vi "Pcre2NextMatch8.vi"(8 "error in":errorcluster, 11 "pMatchData":u64 format="%.0x") -> (0 "error out":errorcluster, 1 "GlobalOptions":u32 format="%.0x", 2 "NextStartOffset":u64, 3 "pMatchData":u64 format="%.0x", 5 "ContinueMatch?":bool)   [LabVIEW 2021, in "libpcre2-8.lvlib"]
uses:
  libpcre2-8.lvlib
  libpcre2-8-x32.dll
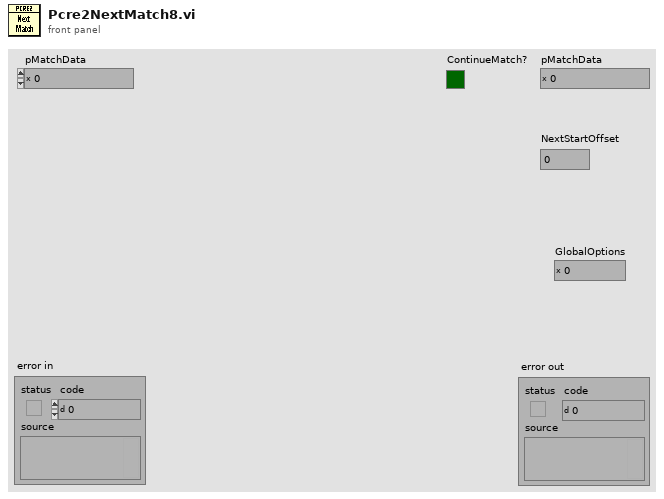
[diagram p1: front panel]
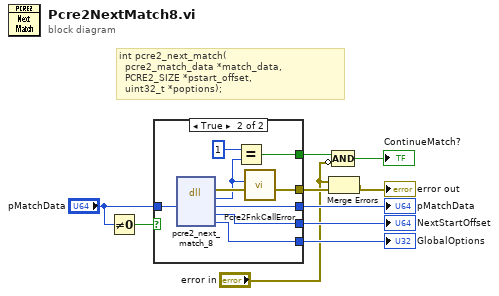
[diagram p0: block diagram]
diagram:
  # "int pcre2_next_match(\n  pcre2_match_data *match_data, \n  PCRE2_SIZE *pstart_offset, \n  uint32_t *poptions);"
  n1 = Not Equal To 0?(x="pMatchData") -> (x != 0?=w6:bool)
  n2 = case shown="True" w6 {
    tunnel: [_ w19] -> w3
    tunnel: "pMatchData" -> [_ w17]
    tunnel: [_ w16] -> w10
    tunnel: [_ w13] -> w5
    tunnel: [_ w12] -> w9
    tunnel: [_ w11] -> w8
    frame False {
    }
    frame True {
      n3 = dll-call lib="libpcre2-8-x*.dll" fn="pcre2_next_match_8"("match_data"=w17) -> (error out=w18:errorcluster, "result"=w15:i32, "match_data"=w16:u64, "pstart_offset"=w12:u64, "poptions"=w11:u32)  [unwired: 5 in, 1 out]
      n4 = Equal?(x=1, y=w15) -> (x = y?=w13:bool)
      n5 = call "Pcre2FnkCallError.vi"("error in"=w18, "ErrorCode"=w15) -> ("error out"=w19:errorcluster)  [unwired: 9 in]
    }
  }
  "pMatchData" <- w10
  "NextStartOffset" <- w9
  "GlobalOptions" <- w8
  n6 = Merge Errors("error in", w3) -> (→"error out":errorcluster)
  n7 = Compound Arithmetic op=AND(w5, invert "error in") -> (→"ContinueMatch?":bool)
